vi "Color row of table.vi"(6 "Edit Line":dbl, 9 "Number of Columns":i32, 10 "Color":u32, 11 "Table in":refnum<vi>) -> (3 "Table out":refnum<vi>)   [LabVIEW 2011]
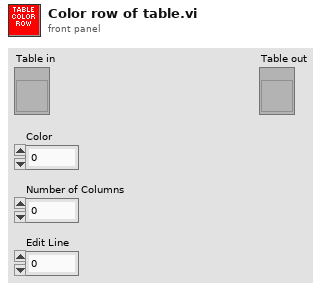
[diagram p1: front panel]
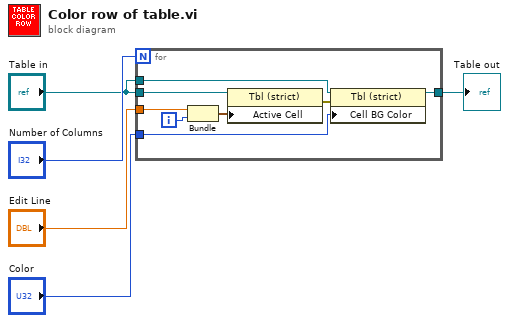
[diagram p0: block diagram]
diagram:
  n1 = for {
    N: "Number of Columns" -> [_]
    tunnel: "Edit Line" -> [w10]
    tunnel: "Color" -> [w9]
    tunnel: "Table in" -> [w8]
    tunnel: "Table in" -> [w7]
    tunnel: [w6] -> w1
    i -> [w12]
    n2 = Bundle("Edit Line"=w10, w12) -> (w13:cluster{"Edit Line":dbl, i32})  [unwired: 1 in]
    n3 = property on="Property Node" class="Tbl (strict)"(reference=w8, "Active Cell"=w13) -> (error out=w11:errorcluster)  [unwired: 1 in, 1 out]
    n4 = property on="Property Node" class="Tbl (strict)"(reference=w7, error in=w11, "Cell BG Color"=w9) -> (reference out=w6:refnum<vi>)  [unwired: 1 out]
  }
  "Table out" <- w1
